vi "Jaccard kNN1.vi"() -> ()   [LabVIEW 2014]
panel:
  out "LCS/min (Lsample,Lknown)":dbl[][](array[numeric])
  out "Distance values (LCS)":dbl[][](array[numeric])
  in  "All data in 2":string[][](array[string])=array2046x3[6138 elements]
  out "size(s)":i32
  out "accuracy":string[][](array[string])
  out "Results":string[][](array[string])
  out "Training data (K)":string[][](array[string])
  out "test data K-1":string[][](array[string])
  in  "K folds K":i32=10
  out "K folds data":string[][](array[string])
  out "Assigned using LCS (enhanced)":string[][](array[string])
  out "Assigned using LCS":string[][](array[string])
  in  "class labels for training data":string[](array[string])
  in  "kNN k":i32=5
  in  "training data (cluster centers)":string[](array[string])
  in  "test data (patterns in)":string[](array[string])=["0 4 0", "4 0 4", "0 4 0", "4 0 4", "0 4 0", "4 0 4", "0 4 0", "4 0 -2", "0 -2 3", "-2 3 0", "3 0 3", "0 3 0", "3 0 4", "0 4 0", "-2 0 1", "0 1 0", "1 0 -4", "0 -4 4", "-2 2 0", "2 0 -1", "0 -1 -4", "-1 -4 1", "-4 1 0", "1 0 3", "0 3 0", "-1 0 -1", "0 -1 2", "0 -1 1", "-1 1 0", "1 0 4", "0 4 0", "4 0 3", "0 3 -2", "3 -2 0", "-2 0 -2", "0 -2 3", "-2 3 -2", "3 -2 0", "-2 0 4", "0 4 0", "4 0 -2", "0 -2 2", "2 -1 0", "-1 0 4", "0 4 0", "4 0 2", "0 2 0", "2 0 -2", "0 -2 0", "1 -1 0", "-1 0 3", "0 3 0", "3 0 -4", "0 -4 4", "-4 4 -4", "4 -4 0", "2 -1 0", "-1 0 3", "0 3 -2", "3 -2 0", "-2 0 -3", "0 -3 0", "-3 0 3", "0 3 0", "3 0 -3", "0 -3 0", "0 4 0", "4 0 4", "0 4 -4", "4 -4 1", "-4 1 -1", "1 -1 0", "-1 0 -3", "0 -3 0", "-3 0 1", "0 1 -4", "1 -4 1", "-4 1 0", "1 0 4", "0 4 0", "4 0 -4", "0 -4 0", "-4 0 -4", "0 -4 4", "-4 4 -4", "4 -4 1", "0 -4 1", "-4 1 0", "1 0 -4", "0 -4 4", "0 4 0", "4 0 -2", "0 -2 2", "-2 2 -2", "2 -2 2", "-2 2 -2", "2 -2 2", "-2 2 -1", "2 -1 0", "-1 0 4", "0 4 0", "4 0 2", "0 2 0", "2 0 4", "0 4 0", "4 0 2", "0 2 -2", "2 -2 0", "-2 0 4", "1 0 -1", "0 -1 0", "-1 0 -1", "0 -1 0", "-1 0 1", "0 1 -1", "-2 2 -2", "2 -2 3", "1 0 -1", "0 -1 0", "-1 0 -1", "0 -1 2", "-1 2 0", "2 0 2", "0 2 -2", "2 -2 0", "-2 0 -4", "0 -4 0", "-2 2 0", "2 0 3", "0 3 -2", "3 -2 2", "1 -1 0", "-1 0 3", "0 4 0", "-2 0 1", "0 1 -4", "1 -4 0", "-4 0 -3", "0 -3 0", "1 0 -1", "0 -1 2", "-1 2 -1", "2 -1 1", "-1 1 -4", "-2 0 -1", "0 -1 1", "0 3 0", "3 0 3", "0 3 0", "3 0 3", "0 3 -2", "-4 0 -4", "0 -4 4", "0 4 0", "4 0 -4", "0 -4 0", "-4 0 -4", "-2 2 0", "2 0 4", "0 4 -4", "4 -4 0", "-4 0 2", "0 2 -2"]
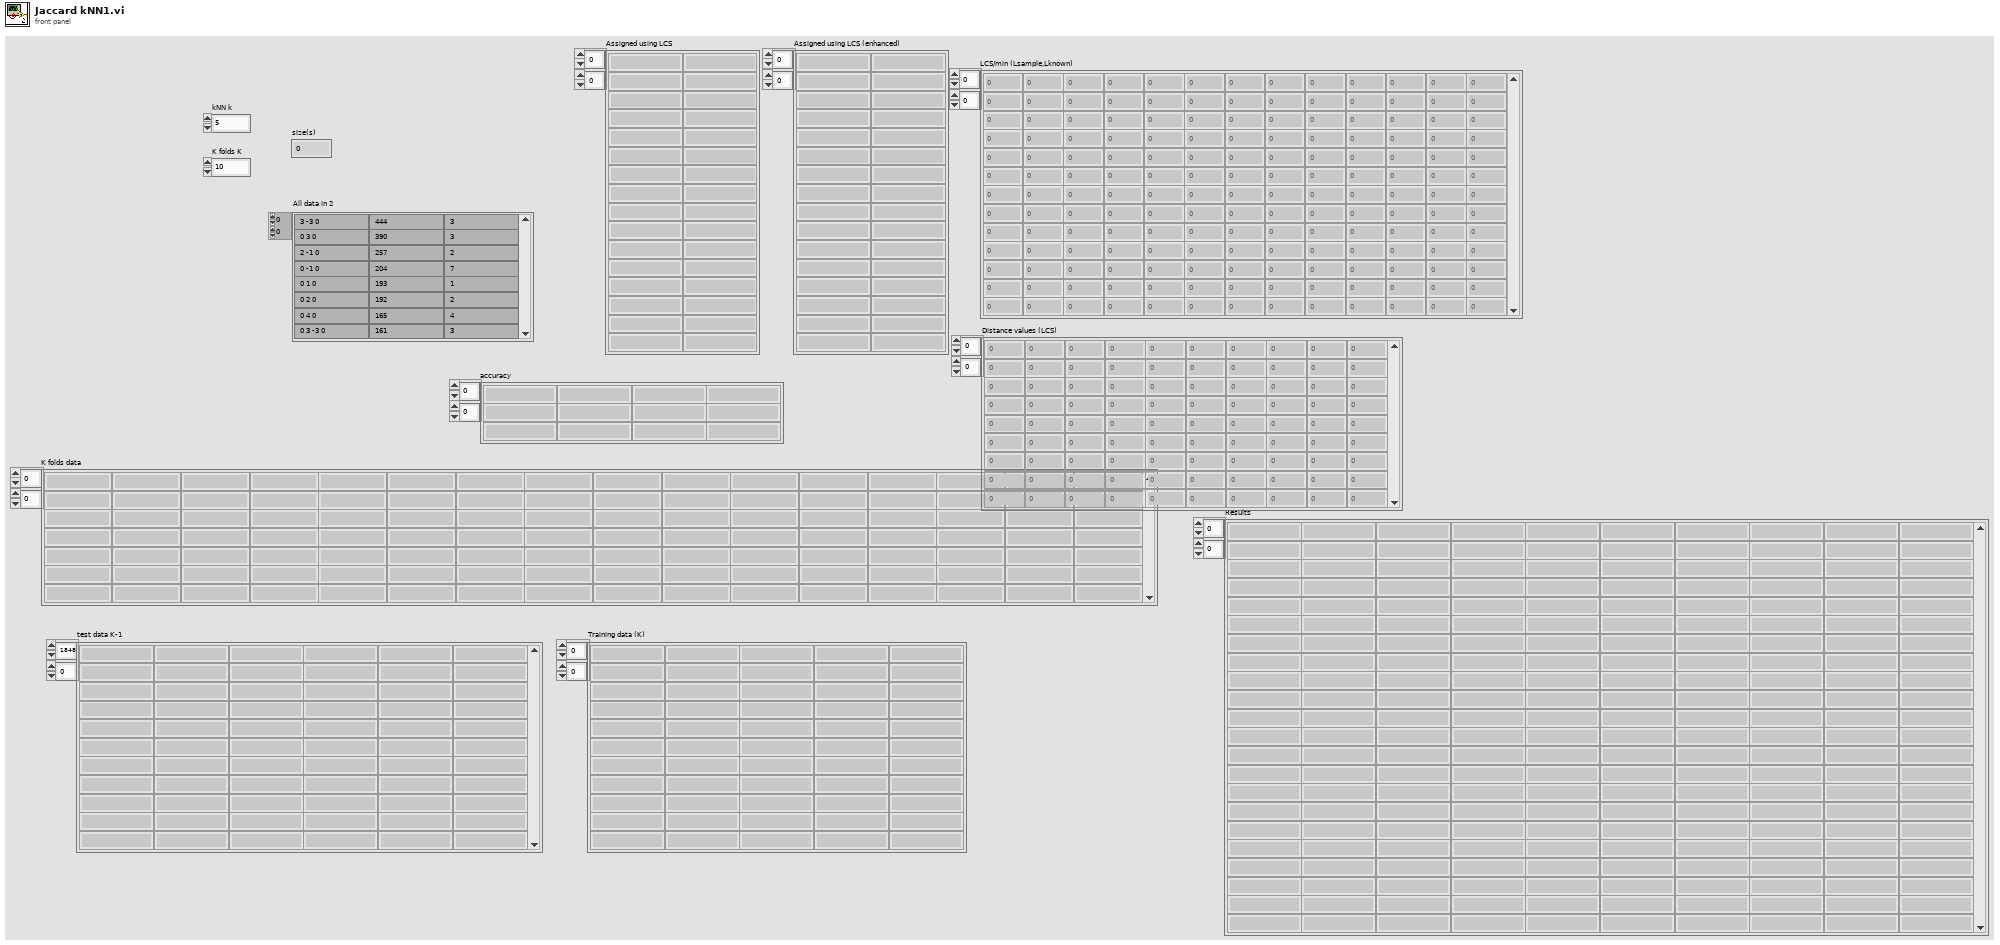
[diagram p1: front panel]
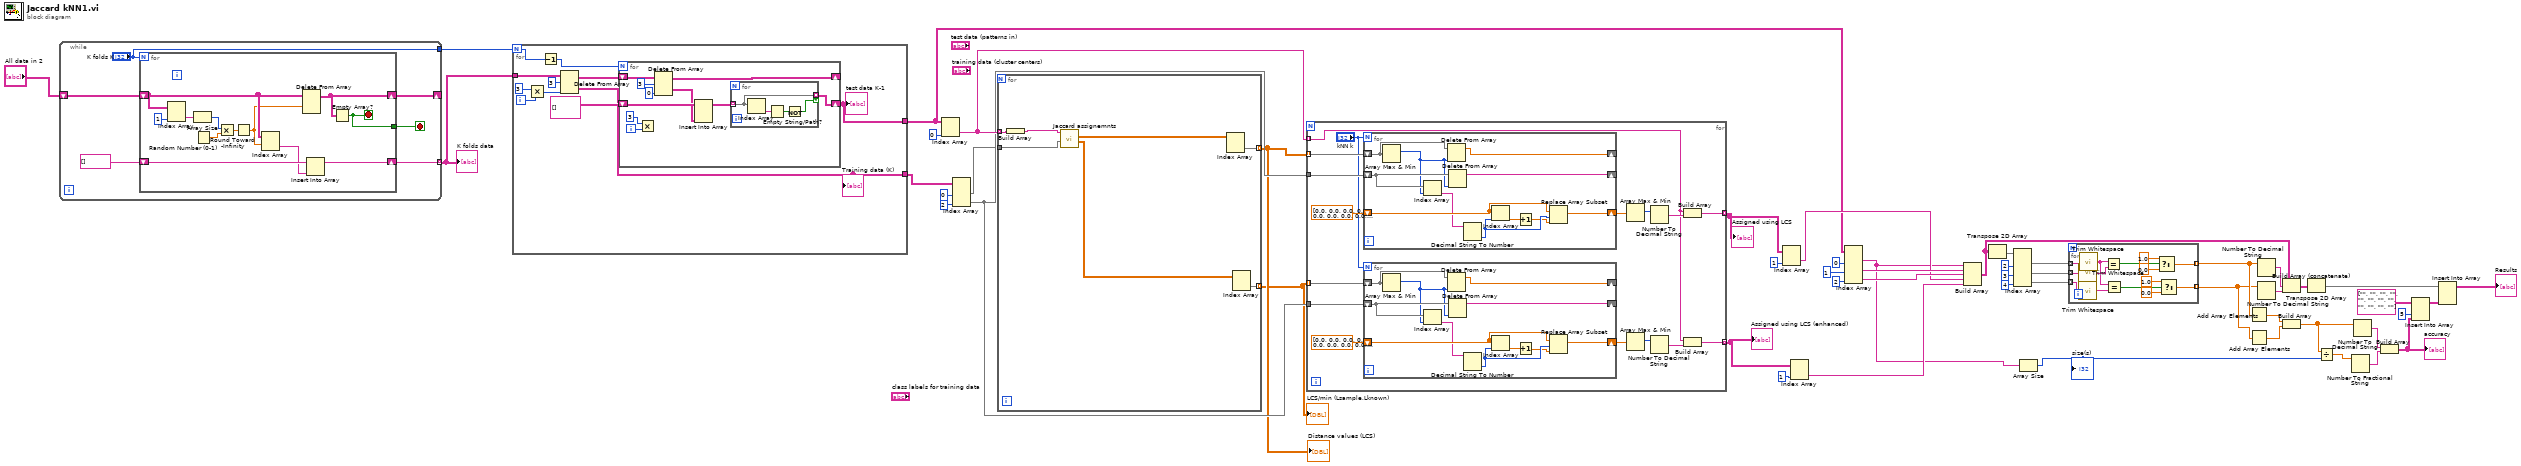
[diagram p0: block diagram]
diagram:
  n1 = while {
    shift-right: [w54] -> _
    shift-left: "All data in 2" -> [w55]
    tunnel: [w56] -> w51 mode=indexing
    tunnel: ["K folds K"] -> w50
    stop <- w53 stop-if-true
    n2 = for {
      N: "K folds K" -> [_]
      shift-right: [w62] -> w56
      shift-left: string[] [] ("all rows 2") -> [w69]
      shift-right: [w60] -> w54
      shift-left: w55 -> [w61]
      tunnel: [w59] -> w53
      stop <- w59 stop-if-true
      n3 = Index Array(array=w61, index (col)=1 ("disabled index (col)")) -> (element=w65:string[])  [unwired: 1 in]
      n4 = Array Size(array=w65) -> (size(s)=w66:i32)
      n5 = Random Number (0-1)() -> (number: 0 to 1=w67:dbl)
      n6 = Multiply(x=w66, y=w67) -> (x*y=w68:dbl)
      n7 = Round Toward -Infinity(1:w68) -> (0:w58:dbl)
      n8 = Index Array(array=w61, index (row)=w58) -> (element=w63:string[])  [unwired: 1 in]
      n9 = Delete From Array(array=w61, index (row)=w58) -> (array with subset deleted=w60:string[][])  [unwired: 2 in, 1 out]
      n10 = Insert Into Array(array=w69, new element=w63) -> (w62:string[])  [unwired: 1 in]
      n11 = Empty Array?(array=w60) -> (empty?=w59:bool)
    }
  }
  "K folds data" <- w51
  n12 = for {
    N: w50 -> [w73]
    tunnel: w51 -> [w80]
    tunnel: [w71] -> w11
    tunnel: [w70] -> w7
    i -> [w78]
    n13 = Multiply(x=3, y=w78) -> (x*y=w76:i32)
    n14 = Decrement(x=w73) -> (x-1=w72:i32)
    n15 = Delete From Array(array=w80, length=3, index (col)=w76) -> (deleted portion=w71:string[][], array with subset deleted=w75:string[][])  [unwired: 1 in]
    "Training data (K)" <- w71
    n16 = for {
      N: w72 -> [_]
      shift-right: [w81] -> w70
      shift-left: string[][] [] ("all rows 2") -> [w89]
      shift-right: [w84] -> _
      shift-left: w75 -> [w90]
      i -> [w86]
      n17 = Multiply(x=3, y=w86) -> ()  [unwired: 1 out]
      n18 = Delete From Array(array=w90, length=3 ("index (col)"), index (col)=0 ("disabled index (col)")) -> (deleted portion=w88:string[][], array with subset deleted=w84:string[][])  [unwired: 1 in]
      n19 = Insert Into Array(array=w89, new element=w88) -> (w82:string[][])  [unwired: 2 in]
      n20 = for {
        tunnel: w82 -> [w93] mode=indexing
        tunnel: [w93] -> w81 mode=indexing if=w94
        n21 = Index Array(array=w93) -> (element=w92:string)  [unwired: 1 in]
        n22 = Empty String/Path?(string/path=w92) -> (empty?=w91:bool)
        n23 = Not(x=w91) -> (.not. x?=w94:bool)
      }
    }
    "test data K-1" <- w70
  }
  n24 = Index Array(array=w7, index (col)=0 ("disabled index (col)")) -> (element=w13:string[])  [unwired: 1 in]
  n25 = Index Array(array=w11, index (col) #1=0 ("disabled index (col)"), index (col) #2=2 ("index (col)")) -> (element #1=w8:string[], element #2=w9:string[])  [unwired: 2 in]
  n26 = for {
    tunnel: w13 -> [w101] mode=indexing
    tunnel: w8 -> [w97]
    tunnel: [w100] -> w2 mode=indexing
    tunnel: [w99] -> w1 mode=indexing
    n27 = Build Array(w101) -> (w98:string[])
    n28 = call "Jaccard assignemnts.vi"("cluster centers in"=w97, "patterns in"=w98) -> ("distance values out enhanced"=w95:dbl[][], "distance values out"=w96:dbl[][])  [unwired: 8 in]
    n29 = Index Array(array=w96) -> (element=w100:dbl[])  [unwired: 2 in]
    n30 = Index Array(array=w95) -> (element=w99:dbl[])  [unwired: 2 in]
  }
  "Distance values (LCS)" <- w2
  "LCS/min (Lsample,Lknown)" <- w1
  n31 = for {
    tunnel: w13 -> [w107] mode=indexing
    tunnel: w2 -> [w117] mode=indexing
    tunnel: w9 -> [w116]
    tunnel: w1 -> [w106] mode=indexing
    tunnel: w9 -> [w105]
    tunnel: [w104] -> w20 mode=indexing
    tunnel: [w103] -> w16 mode=indexing
    n32 = for {
      N: "kNN k" -> [_]
      shift-right: [w136] -> _
      shift-left: w117 -> [w139]
      shift-right: [w135] -> _
      shift-left: w116 -> [w138]
      shift-right: [w130] -> w113
      shift-left: dbl[] [0.0, 0.0, 0.0, 0.0, 0.0, 0.0, 0.0, 0.0, 0.0, 0.0, 0.0, 0.0] -> [w131]
      n33 = Array Max & Min(array=w139) -> (max index (indices)=w137:i32)  [unwired: 3 out]
      n34 = Index Array(array=w138, index=w137) -> (element=w129:string)
      n35 = Delete From Array(array=w139, index=w137) -> (array with subset deleted=w136:dbl[])  [unwired: 1 in, 1 out]
      n36 = Delete From Array(array=w138, index=w137) -> (array with subset deleted=w135:string[])  [unwired: 1 in, 1 out]
      n37 = Decimal String To Number(string=w129) -> (number=w134:i32)  [unwired: 2 in, 1 out]
      n38 = Index Array(array=w131, index=w134) -> (element=w132:dbl)
      n39 = Increment(x=w132) -> (x+1=w133:dbl)
      n40 = Replace Array Subset(array=w131, new element=w133, index=w134) -> (w130:dbl[])
    }
    n41 = for {
      N: "kNN k" -> [_]
      shift-right: [w125] -> _
      shift-left: w106 -> [w128]
      shift-right: [w124] -> _
      shift-left: w105 -> [w127]
      shift-right: [w119] -> w110
      shift-left: dbl[] [0.0, 0.0, 0.0, 0.0, 0.0, 0.0, 0.0, 0.0, 0.0, 0.0, 0.0, 0.0] -> [w120]
      n42 = Array Max & Min(array=w128) -> (max index (indices)=w126:i32)  [unwired: 3 out]
      n43 = Index Array(array=w127, index=w126) -> (element=w118:string)
      n44 = Delete From Array(array=w128, index=w126) -> (array with subset deleted=w125:dbl[])  [unwired: 1 in, 1 out]
      n45 = Delete From Array(array=w127, index=w126) -> (array with subset deleted=w124:string[])  [unwired: 1 in, 1 out]
      n46 = Decimal String To Number(string=w118) -> (number=w123:i32)  [unwired: 2 in, 1 out]
      n47 = Index Array(array=w120, index=w123) -> (element=w121:dbl)
      n48 = Increment(x=w121) -> (x+1=w122:dbl)
      n49 = Replace Array Subset(array=w120, new element=w122, index=w123) -> (w119:dbl[])
    }
    n50 = Array Max & Min(array=w113) -> (max index (indices)=w114:i32)  [unwired: 3 out]
    n51 = Array Max & Min(array=w110) -> (max index (indices)=w109:i32)  [unwired: 3 out]
    n52 = Number To Decimal String(number=w114) -> (decimal integer string=w112:string)  [unwired: 1 in]
    n53 = Number To Decimal String(number=w109) -> (decimal integer string=w111:string)  [unwired: 1 in]
    n54 = Build Array(w107, w112) -> (w104:string[])
    n55 = Build Array(w107, w111) -> (w103:string[])
  }
  "Assigned using LCS" <- w20
  "Assigned using LCS (enhanced)" <- w16
  n56 = Index Array(array=w20, index (col)=1 ("disabled index (col)")) -> (element=w18:string[])  [unwired: 1 in]
  n57 = Index Array(array=w16, index (col)=1 ("disabled index (col)")) -> (element=w15:string[])  [unwired: 1 in]
  n58 = Index Array(array=w7, index (col) #1=0 ("disabled index (col)"), index (col) #2=1 ("index (col)"), index (col) #3=2 ("index (col)")) -> (element #1=w5:string[], element #2=w23:string[], element #3=w22:string[])  [unwired: 3 in]
  n59 = Build Array(w5, w23, w22, w18, w15) -> (w6:string[][])
  n60 = Transpose 2D Array(2D array=w6) -> (transposed array=w41:string[][])
  n61 = Index Array(array=w41, index (col) #1=2 ("disabled index (col)"), index (col) #2=3 ("index (col)"), index (col) #3=4 ("index (col)")) -> (element #1=w44:string[], element #2=w43:string[], element #3=w42:string[])  [unwired: 3 in]
  n62 = Array Size(array=w5) -> (size(s)=w4:i32)
  "size(s)" <- w4
  n63 = for {
    tunnel: w44 -> [w145] mode=indexing
    tunnel: w43 -> [w144] mode=indexing
    tunnel: w42 -> [w143] mode=indexing
    tunnel: [w147] -> w26 mode=indexing
    tunnel: [w146] -> w25 mode=indexing
    n64 = call <vilib>:"Trim Whitespace.vi"("string"=w144) -> ("trimmed string"=w142:string)  [unwired: 1 in]
    n65 = call <vilib>:"Trim Whitespace.vi"("string"=w143) -> ("trimmed string"=w141:string)  [unwired: 1 in]
    n66 = call <vilib>:"Trim Whitespace.vi"("string"=w145) -> ("trimmed string"=w140:string)  [unwired: 1 in]
    n67 = Equal?(x=w140, y=w142) -> (x = y?=w153:bool)
    n68 = Equal?(x=w140, y=w141) -> (x = y?=w148:bool)
    n69 = Select(t=1.0, s=w153, f=0.0) -> (s? t:f=w147:dbl)
    n70 = Select(t=1.0, s=w148, f=0.0) -> (s? t:f=w146:dbl)
  }
  n71 = Add Array Elements(numeric array=w26) -> (sum=w27:dbl)
  n72 = Add Array Elements(numeric array=w25) -> (sum=w28:dbl)
  n73 = Number To Decimal String(number=w26) -> (decimal integer string=w40:string[])  [unwired: 1 in]
  n74 = Number To Decimal String(number=w25) -> (decimal integer string=w39:string[])  [unwired: 1 in]
  n75 = Build Array (concatenate)(w6, w40, w39) -> (w38:string[][])
  n76 = Build Array(w27, w28) -> (w29:dbl[])
  n77 = Transpose 2D Array(2D array=w38) -> (transposed array=w24:string[][])
  n78 = Divide(x=w29, y=w4) -> (x/y=w30:dbl[])
  n79 = Number To Fractional String(number=w30) -> (F-format string=w32:string[])  [unwired: 3 in]
  n80 = Number To Decimal String(number=w29) -> (decimal integer string=w31:string[])  [unwired: 1 in]
  n81 = Build Array(w31, w32) -> (w36:string[][])
  "accuracy" <- w36
  n82 = Insert Into Array(array=string[][] [["", "", "", "", "", ""], ["", "", "", "", "", ""]] ("appended array 3"), index (col)=5 ("disabled index (col)"), new element=w36) -> (w35:string[][])  [unwired: 1 in]
  n83 = Insert Into Array(array=w24, new element=w35) -> (→"Results":string[][])  [unwired: 2 in]
